vi "exercise6_readAI_samples.vi"() -> ()   [LabVIEW 2018]
uses:
  <vilib>/DAQmx/read.llb/DAQmx Read (Analog Wfm 1Chan NSamp).vi
  <vilib>/DAQmx/create/channels.llb/DAQmx Create Channel (AI-Voltage-Basic).vi
  <vilib>/DAQmx/configure/timing.llb/DAQmx Timing (Sample Clock).vi
  <vilib>/DAQmx/miscellaneous.llb/DAQmx Fill In Error Info.vi
panel:
  in  "maximum value":dbl=5.0
  in  "minimum value":dbl=-5.0
  in  "sample mode":i32(ring)=10123 items=["Finite Samples"=10178, "Continuous Samples"=10123, "Hardware Timed Single Point"=12522]
  in  "samples per channel":i32=150000
  in  "rate":dbl=15000.0
  out "error out":errorcluster
  out "Waveform Graph":waveform(dbl)(graph)
  out "Waveform Chart":waveform(dbl)(graph)
  in  "NI_channels":tag="Dev1/ai0"
  # "CANAL 0"
  # "CANAL 0"
  # "ACQUIRE SIGNAL"
  # "CHANNEL CONFIG"
  # "SAMPLING CONFIG"
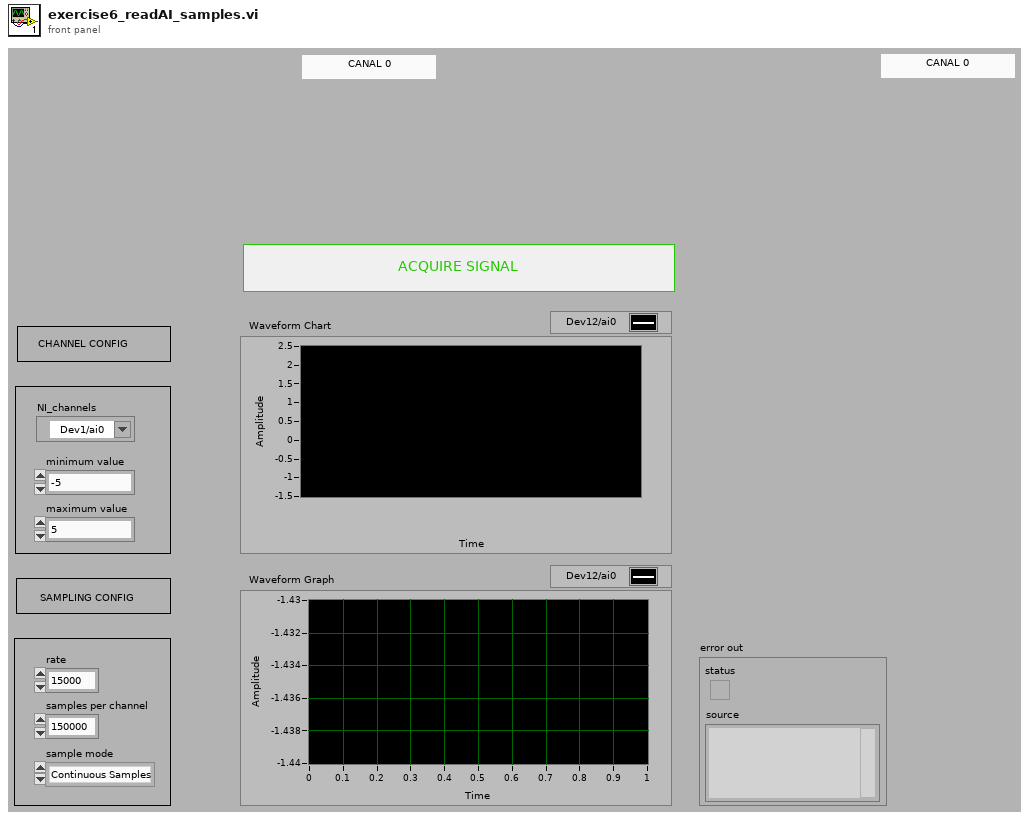
[diagram p1: front panel]
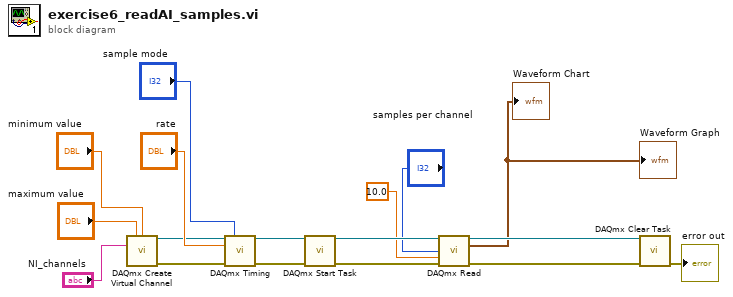
[diagram p0: block diagram]
diagram:
  n1 = call-poly <vilib>:"DAQmx Create Virtual Channel.vi"("maximum value"="maximum value", "minimum value"="minimum value", "physical channels"="NI_channels") -> ("task out"=w15:refnum<k21>, "error out"=w14:errorcluster)  [unwired: 11 in]
  n2 = call-poly <vilib>:"DAQmx Timing.vi"("task/channels in"=w15, "sample mode"="sample mode", "rate"="rate", "error in"=w14) -> ("task out"=w10:refnum<k21>, "error out"=w9:errorcluster)  [unwired: 10 in]
  n3 = call <vilib>:"DAQmx Start Task.vi"("task/channels in"=w10, "error in"=w9) -> ("task out"=w7:refnum<k21>, "error out"=w8:errorcluster)  [unwired: 12 in]
  n4 = call-poly <vilib>:"DAQmx Read.vi"("task/channels in"=w7, "number of samples per channel"="samples per channel", "timeout"=10.0, "error in"=w8) -> ("task out"=w5:refnum<k21>, "data"=→"Waveform Graph" →"Waveform Chart":waveform(dbl), "error out"=w6:errorcluster)  [unwired: 9 in]
  n5 = call <vilib>:"DAQmx Clear Task.vi"("task in"=w5, "error in"=w6) -> ("error out"=→"error out":errorcluster)  [unwired: 13 in]
